vi "stable error and currents.vi"(0 "Charge State":dbl=7.0, 1 "ss ratio 2":u16(ring) items=["other", "36Cl"], 2 "ss ratio":dbl, 5 "Stable Current 1":dbl, 7 "Tails":dbl, 9 "Stable Current 2":dbl, 11 "Live Time":dbl, 13 "deadtime":dbl) -> (4 "Delta stable current value":dbl, 6 "Stable Counts":dbl)   [LabVIEW 2016]
doc: "This vi inputs the values need to calculate the error and q value for the stable currents and returns those values"
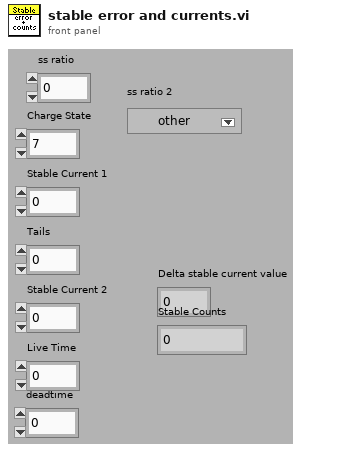
[diagram p1: front panel]
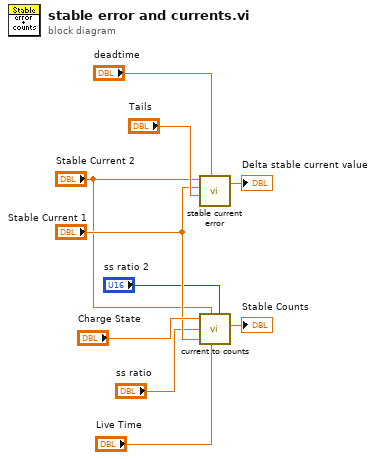
[diagram p0: block diagram]
diagram:
  n1 = call "stable current error.vi"("Stable Current 2"="Stable Current 2", "Stable Current 1"="Stable Current 1", "Tails"="Tails", "deadtime"="deadtime") -> ("Delta stable current value"=→"Delta stable current value":dbl)  [unwired: 1 in, 1 out]
  n2 = call "current to counts.vi"("Charge State"="Charge State", "Stable Current 2"="Stable Current 2", 2:"ss ratio"="ss ratio", "Stable Current 1"="Stable Current 1", "Live Time"="Live Time", 5:"ss ratio"="ss ratio 2") -> ("Stable Counts"=→"Stable Counts":dbl)  [unwired: 4 in]
